vi "temperature_Vcc.vi"(8 "error in (no error)":errorcluster, 10 "Address 2":u32=3, 11 "IP address":string="192.168.10.23") -> (0 "error out":errorcluster={"status"=TRUE, "code"=56, "source"="UDP Read in UDP.vi->flash.vi"}, 2 "Vcc_int[mV]":dbl=985.107421875, 3 "Tc[℃]":dbl=51.80067749023442)   [LabVIEW 2017]
panel:
  out "Out 9":u16=1345 format="%.0x"
  out "Out 8":u16=84 format="%.0x"
  out "Out 7":u16=1344 format="%.0x"
  out "Out 6":u16=1 format="%.0x"
  out "Out 5":u8=10 format="%.0x"
  out "Out 4":u16=2641 format="%.0x"
  out "Out 3":u16=2560 format="%.0x"
  out "Out 2":u8=26 format="%.0x"
  out "Out":u8=81 format="%.0x"
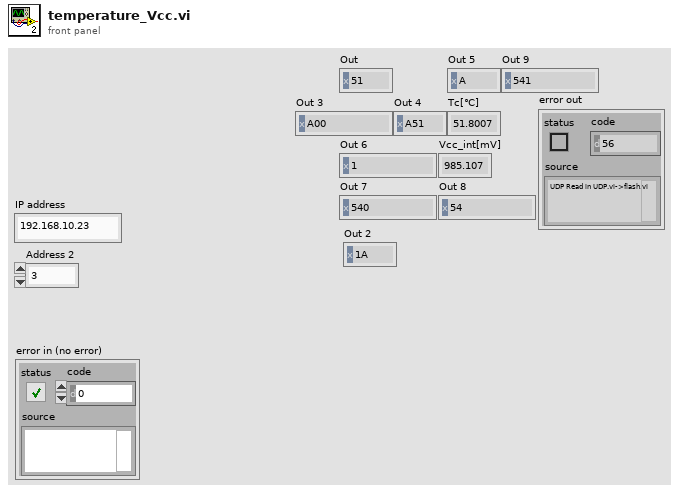
[diagram p1: front panel]
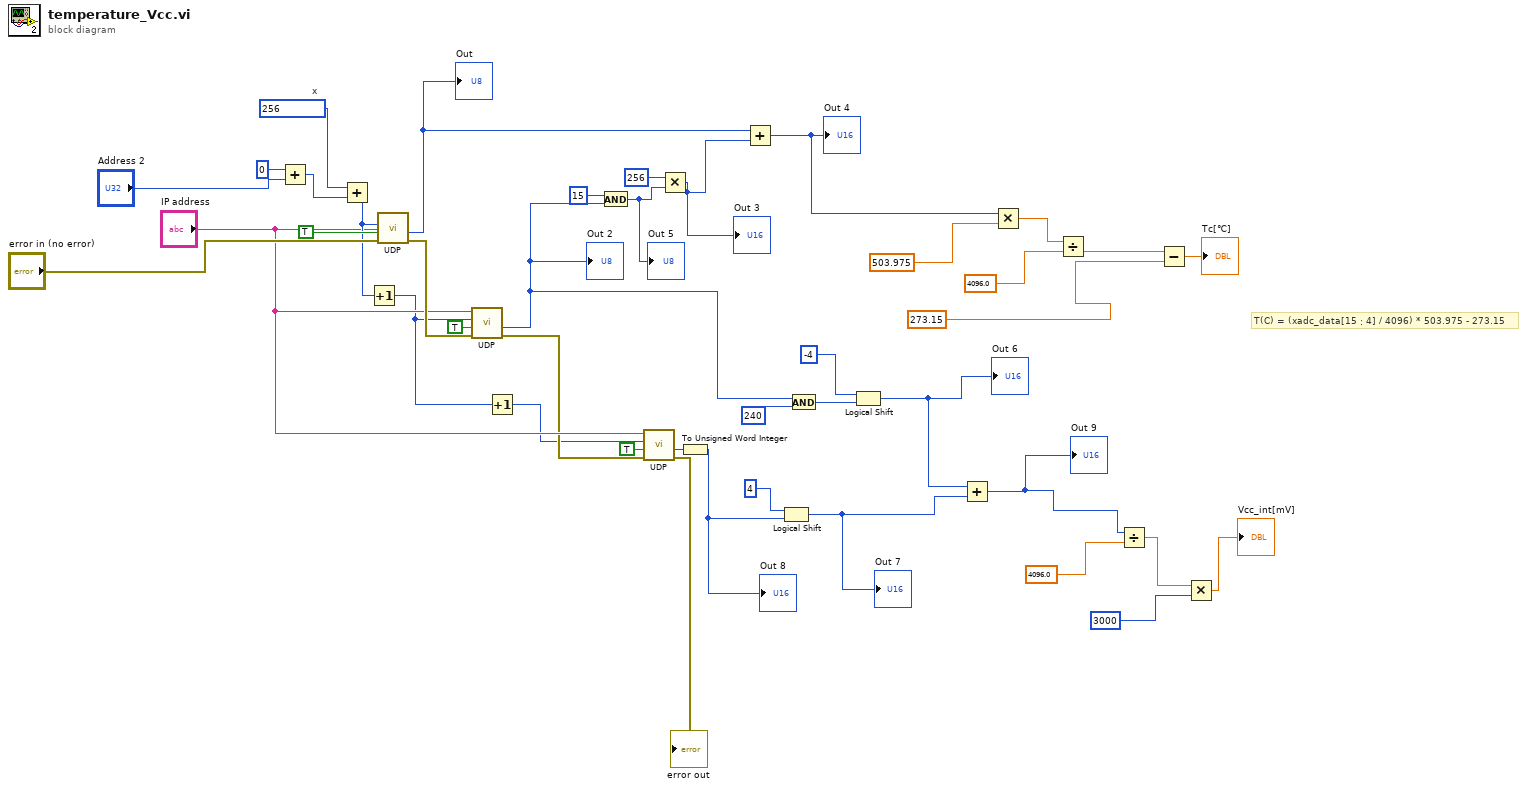
[diagram p0: block diagram]
diagram:
  w40 = u16 256  # x
  # "T(C) = (xadc_data[15：4] / 4096) * 503.975 - 273.15"
  n1 = Add(x=u8 0, y="Address 2") -> (x+y=w37:u32)
  n2 = Add(x=w40, y=w37) -> (x+y=w34:u32)
  n3 = Increment(x=w34) -> (x+1=w8:u32)
  n4 = call "UDP.vi"("error in (no error)"="error in (no error)", "Read (TRUE)"=TRUE, "Address"=w34, "IP address"="IP address") -> ("error out"=w35:errorcluster, "Out"=w29:u8)  [unwired: 5 in]
  "Out" <- w29
  n5 = call "UDP.vi"("error in (no error)"=w35, "Read (TRUE)"=TRUE, "Address"=w8, "IP address"="IP address") -> ("error out"=w19:errorcluster, "Out"=w18:u8)  [unwired: 5 in]
  "Out 2" <- w18
  n6 = Increment(x=w8) -> (x+1=w7:u32)
  n7 = And(x=u8 15, y=w18) -> (x .and. y?=w28:u8)
  "Out 5" <- w28
  n8 = call "UDP.vi"("error in (no error)"=w19, "Read (TRUE)"=TRUE, "Address"=w7, "IP address"="IP address") -> ("error out"=→"error out":errorcluster, "Out"=w9:u8)  [unwired: 5 in]
  n9 = Multiply(x=u16 256, y=w28) -> (x*y=w30:u16)
  "Out 3" <- w30
  n10 = To Unsigned Word Integer(number=w9) -> (unsigned 16bit integer=w6:u16)
  "Out 8" <- w6
  n11 = Add(x=w29, y=w30) -> (x+y=w27:u16)
  "Out 4" <- w27
  n12 = Logical Shift(y=i16 4, x=w6) -> (x << y=w10:u16)
  "Out 7" <- w10
  n13 = And(x=w18, y=u8 240 ("x")) -> (x .and. y?=w16:u8)
  n14 = Logical Shift(y=i16 -4, x=w16) -> (x << y=w13:u8)
  "Out 6" <- w13
  n15 = Add(x=w13, y=w10) -> (x+y=w4:u16)
  "Out 9" <- w4
  n16 = Multiply(x=w27, y=503.975) -> (x*y=w25:dbl)
  n17 = Divide(x=w25, y=4096.0) -> (x/y=w24:dbl)
  n18 = Divide(x=w4, y=4096.0) -> (x/y=w3:dbl)
  n19 = Subtract(x=w24, y=273.15) -> (x-y=→"Tc[℃]":dbl)
  n20 = Multiply(x=w3, y=u16 3000) -> (x*y=→"Vcc_int[mV]":dbl)
